vi "from string 1.0.vi"(8 "error in (no error)":errorcluster, 10 "data":string, 11 "JSON_RPC_Interface configuration in":refnum<class "JSON_RPC_Interface configuration.lvclass">) -> (0 "error out":errorcluster, 3 "JSON_RPC_Interface configuration out":refnum<class "JSON_RPC_Interface configuration.lvclass">)   [LabVIEW 2017, in "JSON_RPC_Interface configuration.lvclass"]
uses:
  JSON_RPC_Interface configuration.lvclass
  <vilib>/NI/Tag Bus Module Framework/channel/TBM channel.lvclass
  Line.ctl
  JSON_RPC_Interface configuration.lvclass/JSON_RPC_Interface configuration.ctl
  <vilib>/NI/Configuration Framework/serializable configuration/NISE_CEF_serializable configuration.lvclass
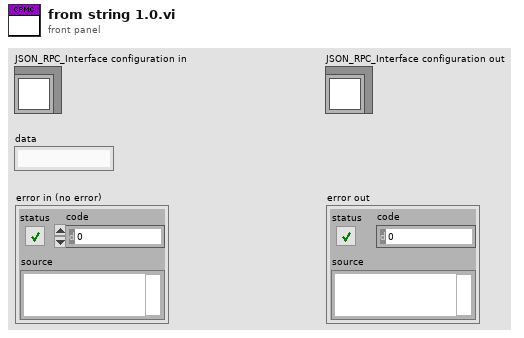
[diagram p1: front panel]
types:
  T1 = typedef "JSON_RPC_Interface configuration.lvclass/Line.ctl" = cluster{"channel":refnum<class "TBM channel.lvclass">}
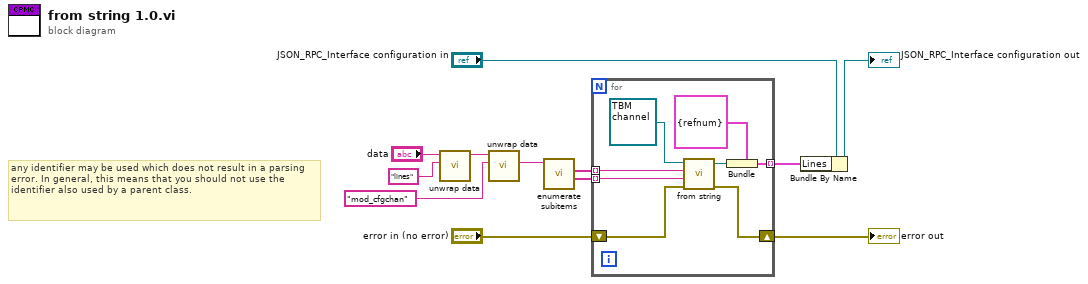
[diagram p0: block diagram]
diagram:
  # "any identifier may be used which does not result in a parsing error. In general, this means that you should not use the identifier also used by a parent class."
  n1 = call <vilib>:"unwrap data.vi"("identifier"="lines" ("additional identifier"), "data to unwrap"="data") -> ("remaining string"=w5:string)  [unwired: 8 in, 1 out]
  n2 = call <vilib>:"unwrap data.vi"("identifier"="mod_cfgchan", "data to unwrap"=w5) -> ("unwrapped data"=w10:string)  [unwired: 8 in, 1 out]
  n3 = call <vilib>:"enumerate subitems.vi"("data to enumerate"=w10) -> ("associated data"=w8:string[], "discovered subitems"=w7:string[])  [unwired: 8 in, 1 out]
  n4 = for {
    shift-right: [w20] -> w12
    shift-left: "error in (no error)" -> [w19]
    tunnel: w7 -> [w18] mode=indexing
    tunnel: w8 -> [w17] mode=indexing
    tunnel: [w13] -> w11 mode=indexing
    n5 = call-dynamic "from string.vi"("error in"=w19, "channel data"=w17, "identifier"=w18, "channel in"=refnum<class "TBM channel.lvclass"> refnum) -> ("error out"=w20:errorcluster, "channel out"=w14:refnum<class "TBM channel.lvclass">)  [unwired: 6 in]
    n6 = Bundle(cluster=T1 {"channel"=refnum} ("Line"), "channel"=w14) -> (w13:T1)
  }
  "error out" <- w12
  n7 = Bundle By Name(cluster="JSON_RPC_Interface configuration in", "Lines"=w11) -> (→"JSON_RPC_Interface configuration out":refnum<class "JSON_RPC_Interface configuration.lvclass">)
